vi "macro_Digital_Or.vi"   [LabVIEW 2019, in "Trajectory_Library.lvlib"]
uses:
  Trajectory_Library.lvlib
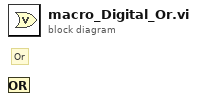
[diagram p0: block diagram]
diagram:
  # "Or"
  n1 = Or() -> ()  [unwired: 2 in, 1 out]
